vi "整理非小号前百位数据.vi"() -> ()   [LabVIEW 2020]
uses:
  <vilib>/Utility/file.llb/Read Delimited Spreadsheet (string).vi
  <vilib>/Utility/file.llb/Write Delimited Spreadsheet (string).vi
panel:
  out "长度":i32
  in  "file path (dialog if empty) 2":path caption="文件路径 （空时为对话框）"
  out "x-y*floor(x/y) 2":i32
  out "1D data":string[](array[string]) caption="一维数据"
  out "all rows":string[][](array[string]) caption="所有行"
  in  "file path (dialog if empty)":path caption="文件路径 （空时为对话框）"
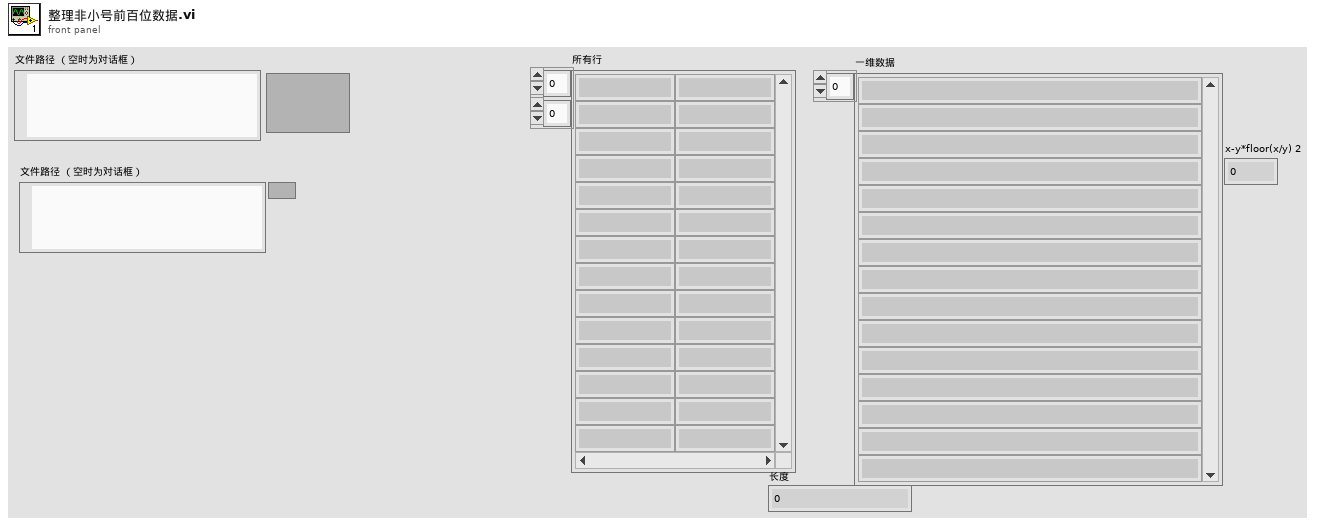
[diagram p1: front panel]
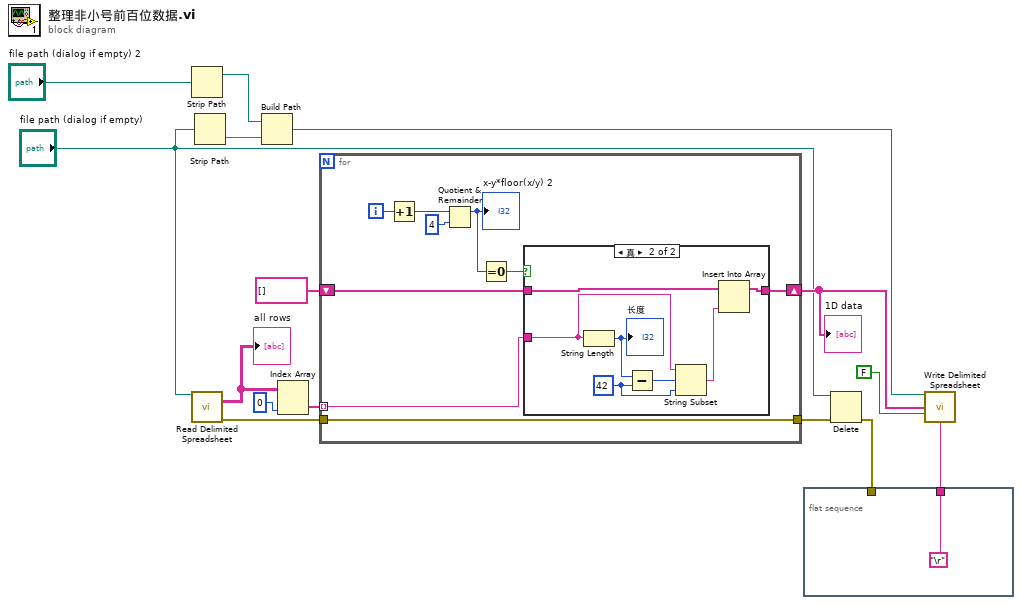
[diagram p0: block diagram]
diagram:
  n1 = Strip Path(path="file path (dialog if empty) 2") -> (stripped path=w7:path)  [unwired: 1 out]
  n2 = call-poly <vilib>:"Read Delimited Spreadsheet.vi"("file path (dialog if empty)"="file path (dialog if empty)") -> ("all rows"=w15:string[][], "error out"=w5:errorcluster)  [unwired: 9 in, 4 out]
  "all rows" <- w15
  n3 = Strip Path(path="file path (dialog if empty)") -> (name=w6:string)  [unwired: 1 out]
  n4 = Build Path(base path=w7, name or relative path=w6) -> (appended path=w11:path)
  n5 = Index Array(array=w15, index (col)=0 ("禁用的索引 (列)")) -> (element=w14:string[])  [unwired: 1 in]
  n6 = for {
    tunnel: w14 -> [w18] mode=indexing
    shift-right: [w17] -> w9
    shift-left: string[] [] -> [w19]
    tunnel: w5 -> [w16]
    tunnel: [w16] -> w4
    i -> [w24]
    n7 = Increment(x=w24) -> (x+1=w23:i32)
    n8 = Quotient & Remainder(x=w23, y=4) -> (x-y*floor(x/y)=w21:i32)  [unwired: 1 out]
    "x-y*floor(x/y) 2" <- w21
    n9 = Equal To 0?(x=w21) -> (x = 0?=w20:bool)
    n10 = case shown="真" w20 {
      tunnel: w19 -> [w25 w32]
      tunnel: w18 -> [_ w27]
      tunnel: [w25 w31] -> w17
      frame False {
      }
      frame True {
        w28 = 42 ("长度（剩余）")
        n11 = String Length(string=w27) -> (length=w30:i32)
        "长度" <- w30
        n12 = Subtract(x=w30, y=w28) -> (x-y=w29:i32)
        n13 = String Subset(string=w27, offset (0)=w29, length (rest)=w28) -> (substring=w26:string)
        n14 = Insert Into Array(array=w32, new element=w26) -> (w31:string[])  [unwired: 1 in]
      }
    }
  }
  "1D data" <- w9
  n15 = flat-sequence {
    tunnel: w2 -> [_]
    tunnel: ["\r"] -> w1
    frame #0 {
    }
  }
  n16 = Delete(path (use dialog)="file path (dialog if empty)", error in=w4) -> (error out=w2:errorcluster)  [unwired: 3 in, 2 out]
  n17 = call-poly <vilib>:"Write Delimited Spreadsheet.vi"("file path (dialog if empty)"=w11, "1D data"=w9, "append to file? (new file:F)"=FALSE, "delimiter (\\t)"=w1) -> ()  [unwired: 10 in, 2 out]
